vi "rs3_MemCopyRGB_IR.vi"(0 "Zimage pointer":u64, 5 "RGB  X, width":i32, 7 "RGB Y, height":i32, 9 "Monochrome(T)/Color(F)":bool, 11 "error in (no error)":errorcluster) -> (4 "Output Array":u8[](array[numeric]), 10 "Length":i32=10, 15 "error out":errorcluster)   [LabVIEW 2017, in "libRealSense3.lvlib"]
doc: "Use this after a getZimage function call, to copy the memory pointed to, into an 2D array in LabVIEW."
uses:
  libRealSense3.lvlib
panel:
  # "RS3_Mem Copy_RGB/IR"
  # "(C) Intel Corp.,  AGJ"
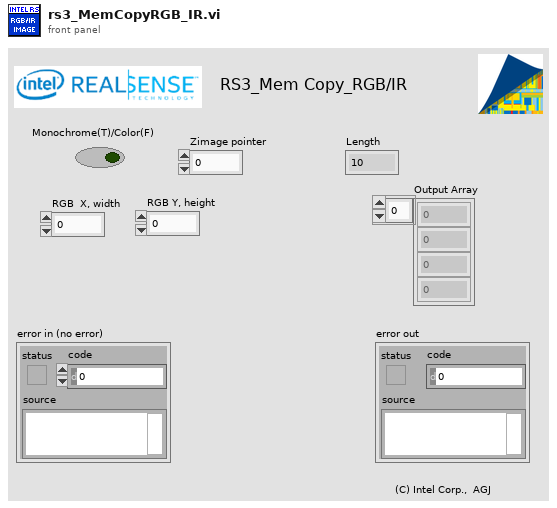
[diagram p1: front panel]
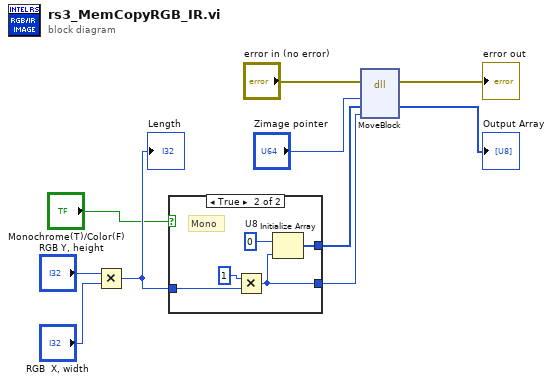
[diagram p0: block diagram]
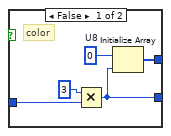
[diagram p2: hidden frame]
diagram:
  n1 = Multiply(x="RGB Y, height", y="RGB  X, width") -> (x*y=w6:i32)
  "Length" <- w6
  n2 = case shown="True" "Monochrome(T)/Color(F)" {
    tunnel: [w12 w19] -> w7
    tunnel: w6 -> [w13 w18]
    tunnel: [w11 w17] -> w5
    frame False {
      w15 = u8 0  # U8
      # "color"
      n3 = Multiply(x=3 ("# of bytes/number"), y=w13) -> (x*y=w11:i32)
      n4 = Initialize Array(w15, w11) -> (w12:u8[])
    }
    frame True {
      w20 = u8 0  # U8
      # "Mono"
      n5 = Multiply(x=1 ("# of bytes/number"), y=w18) -> (x*y=w17:i32)
      n6 = Initialize Array(w20, w17) -> (w19:u8[])
    }
  }
  n7 = dll-call lib="LabVIEW" fn="MoveBlock"(error in="error in (no error)", "Address(Pointer)"="Zimage pointer", "Destination"=w7, "Size"=w5) -> (error out=→"error out":errorcluster, "Destination"=→"Output Array":u8[])  [unwired: 5 in, 1 out]
